vi "Closed Notifier.vi"(11 "Hierarchy (Auto)":string) -> (3 "Closed Notifier":refnum<notifier>)   [LabVIEW 2022 SP3, in "FlexBlocks Support.lvlib"]
uses:
  FlexBlocks Support.lvlib
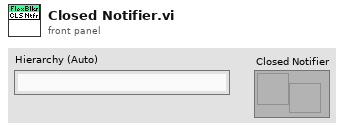
[diagram p1: front panel]
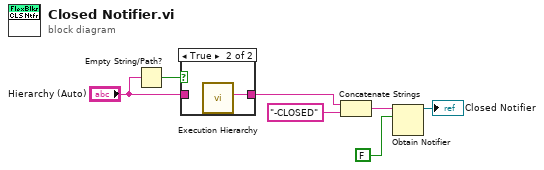
[diagram p0: block diagram]
diagram:
  n1 = Empty String/Path?(string/path="Hierarchy (Auto)") -> (empty?=w6:bool)
  n2 = case shown="True" w6 {
    tunnel: "Hierarchy (Auto)" -> [w8 _]
    tunnel: [w8 w9] -> w4
    frame False {
    }
    frame True {
      n3 = call "Execution Hierarchy.vi"() -> ("Top Level VI Name"=w9:string)  [unwired: 11 in]
    }
  }
  n4 = Concatenate Strings(w4, "-CLOSED" ("string")) -> (w3:string)
  n5 = Obtain Notifier(name (unnamed)=w3, notification data type=FALSE) -> (notifier out=→"Closed Notifier":refnum<notifier>)  [unwired: 2 in, 2 out]
